vi "Scale Matrix.vi"(1 "Matrix":T1 format="%_8f", 4 "Scale Factor":dbl format="%_8f") -> (15 "Scaled Matrix":T1 format="%_8g")   [LabVIEW 2014]
uses:
  <vilib>/Analysis/Matrix/Datatypes/RealMatrix.ctl
  <vilib>/Analysis/baseanly.llb/Real A x B.vi
  <vilib>/Analysis/NI_AALBase.lvlib
  <vilib>/Analysis/Matrix/NI_Matrix.lvlib
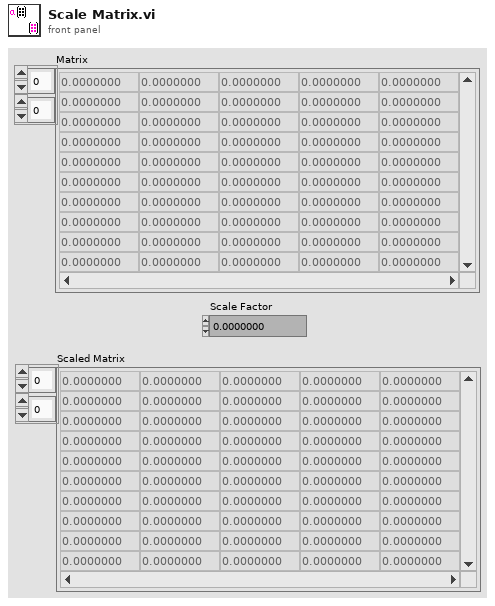
[diagram p1: front panel]
types:
  T1 = typedef "NI_Matrix.lvlib/RealMatrix.ctl" = dbl[][]
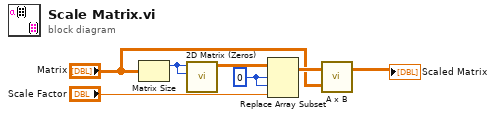
[diagram p0: block diagram]
diagram:
  w5 = 0 ("disabled index (row)")
  n1 = Matrix Size(0:"Matrix") -> (1:w7:i32)  [unwired: 1 out]
  n2 = call "2D Matrix (Zeros).vi"("nCols (1)"=w7, "nRows"=w7) -> ("Real Matrix"=w6:T1)  [unwired: 9 in]
  n3 = Replace Array Subset(array=w6, new element="Scale Factor", index (row)=w5, index (col)=w5) -> (w2:T1)
  n4 = call-poly <vilib>:"A x B.vi"("B"="Matrix", "A"=w2) -> ("A x B"=→"Scaled Matrix":T1)  [unwired: 1 out]
